vi "test1.vi"() -> ()   [LabVIEW 2017]
uses:
  Globals/Global - Configuration Options.vi
panel:
  out "# of Channels":u32=11
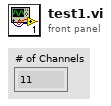
[diagram p1: front panel]
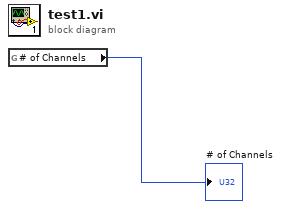
[diagram p0: block diagram]
diagram:
  n1 = global read "Global - Configuration Options.vi" "# of Channels"() -> (→"# of Channels":u32)
